vi "运维调试_采配水V4.vi"() -> ()   [LabVIEW 2016, in "PLC.lvlib"]
uses:
  PLC.lvlib
  control/switch.ctl
  <vilib>/Plasmionique/MB Master/MB_Master/MB_Master.lvclass
  <vilib>/Utility/miscctls.llb/LVPointTypeDef.ctl
  <vilib>/Plasmionique/MB Master/MB_Master_Serial/MB_Master_Serial.lvclass
  C:/Program Files (x86)/National Instruments/LabVIEW 2016/vi.lib/Plasmionique/MB Master/MB_Master/MB_Master.lvclass
  <vilib>/Instr/_visa.llb/VISA Configure Serial Port (Instr).vi
  <vilib>/Plasmionique/MB Master/MB Master.lvlib
panel:
  out "R135":i16 caption="除藻时间"
  in  "R134":u16(ring) caption="除藻工作模式" items=["手动", "自动"]
  in  "R110":u16(ring) caption="反冲洗水体" items=["自来水", "河水"]
  in  "63μm反冲洗阀":bool
  out "R34":u16
  in  "Y21":T1
  out "供水压力":dbl format="%.4f"
  out "R44":u16
  in  "Y31":T1
  out "R111":i16 caption="三级水样池润洗时间"
  in  "三级过滤系统":bool
  out "R104":i16 caption="三级润洗时间"
  out "R103":i16 caption="二级润洗时间"
  out "R107":i16 caption="进气时间"
  out "R43":u16
  in  "Y30":T1
  out "Registers":u16[](array[numeric])
  out "R124":i16 caption="加标回收配水时间"
  out "R42":i16
  in  "Y29":T1
  in  "更新程序":T1
  out "R122":i16 caption="二级自来水清洗时间"
  out "R121":i16 caption="一级自来水清洗时间"
  out "R120":i16 caption="过滤自来水清洗时间"
  out "清洗次数":u16
  out "当前启动泵号":u16(ring) items=["1号泵", "2号泵"]
  out "R116":i16 caption="储水时间"
  in  "R113":u16(ring) caption="水箱储水水体" items=["自来水", "河水"]
  out "R112":i16 caption="二级水样池进样超时"
  out "R31":u16
  out "R30":u16
  out "R29":u16
  out "R28":u16
  out "R27":u16
  out "R26":u16
  out "R25":u16
  out "R24":u16
  out "R23":u16
  out "R22":u16
  out "R21":u16
  out "R20":u16
  out "R19":u16
  out "R18":u16
  out "R17":u16
  out "R16":u16
  out "R15":u16
  out "R14":u16
  out "R13":u16
  out "配水压力":dbl format="%.4f"
  in  "Y18":T1
  in  "Y17":T1
  in  "Y14":T1
  in  "Y13":T1
  in  "Y1":T1
  in  "Y0":T1
  in  "Y12":T1
  in  "Y11":T1
  in  "Y10":T1
  in  "Y9":T1
  in  "Y8":T1
  in  "Y7":T1
  out "X2":bool caption="X1"
  out "采配水版本号":string
  out "R117":i16 caption="清洗频次设定"
  out "通讯故障":bool
  in  "R100":u16(ring) caption="采水泵工作模式" items=["泵1单泵单管路", "泵2单泵单管路", "潜水泵双泵双管路", "自吸泵双泵双管路"]
  out "X10":bool caption="氨氮水样池液位开关SL3"
  out "X9":bool caption="泵2过载报警_KM2"
  out "X8":bool caption="泵1过载报警_KM1"
  out "X7":bool caption="断电检测_PA"
  out "X6":bool caption="门禁开关_AS"
  out "X5":bool caption="烟雾检测_SA"
  out "X4":bool caption="浸水检测_WIA"
  out "X3":bool caption="水流开关_FS"
  out "X1":bool
  out "X0":bool caption="采样池液位开关_SL1"
  out "R109":i16 caption="外部反冲洗时间"
  out "集成报警信息":string
  out "R108":i16 caption="进样超时时间"
  out "R106":i16 caption="排液时间"
  out "R105":i16 caption="常规模式配水时间"
  out "R102":i16 caption="沉淀时间"
  out "R101":i16 caption="一级润洗时间"
  out "R2":i16
  out "R1":i16
  out "多列列表框":i32(listbox)
  in  "Y6":T1
  in  "Y5":T1
  in  "Y4":T1
  in  "Y3":T1
  in  "Y2":T1
  in  "Y16":T1
  in  "Y15":T1
  in  "返回":T1
  in  "参数设置":T1
  in  "单步启动":T1
  in  "启动":T1
  in  "停止":T1
  # "s"
  # "流程计时："
  # "s"
  # "单步计时："
  # "MPa"
  # "配水压力："
  # "MPa"
  # "供水压力："
  # "S"
  # "S"
  # "S"
  # "S"
  # "S"
  # "S"
  # "S"
  # "S"
  # "S"
  # "S"
  # "S"
  # "次"
  # "S"
  # "S"
  # "S"
  # "S"
  # "S"
  # "S"
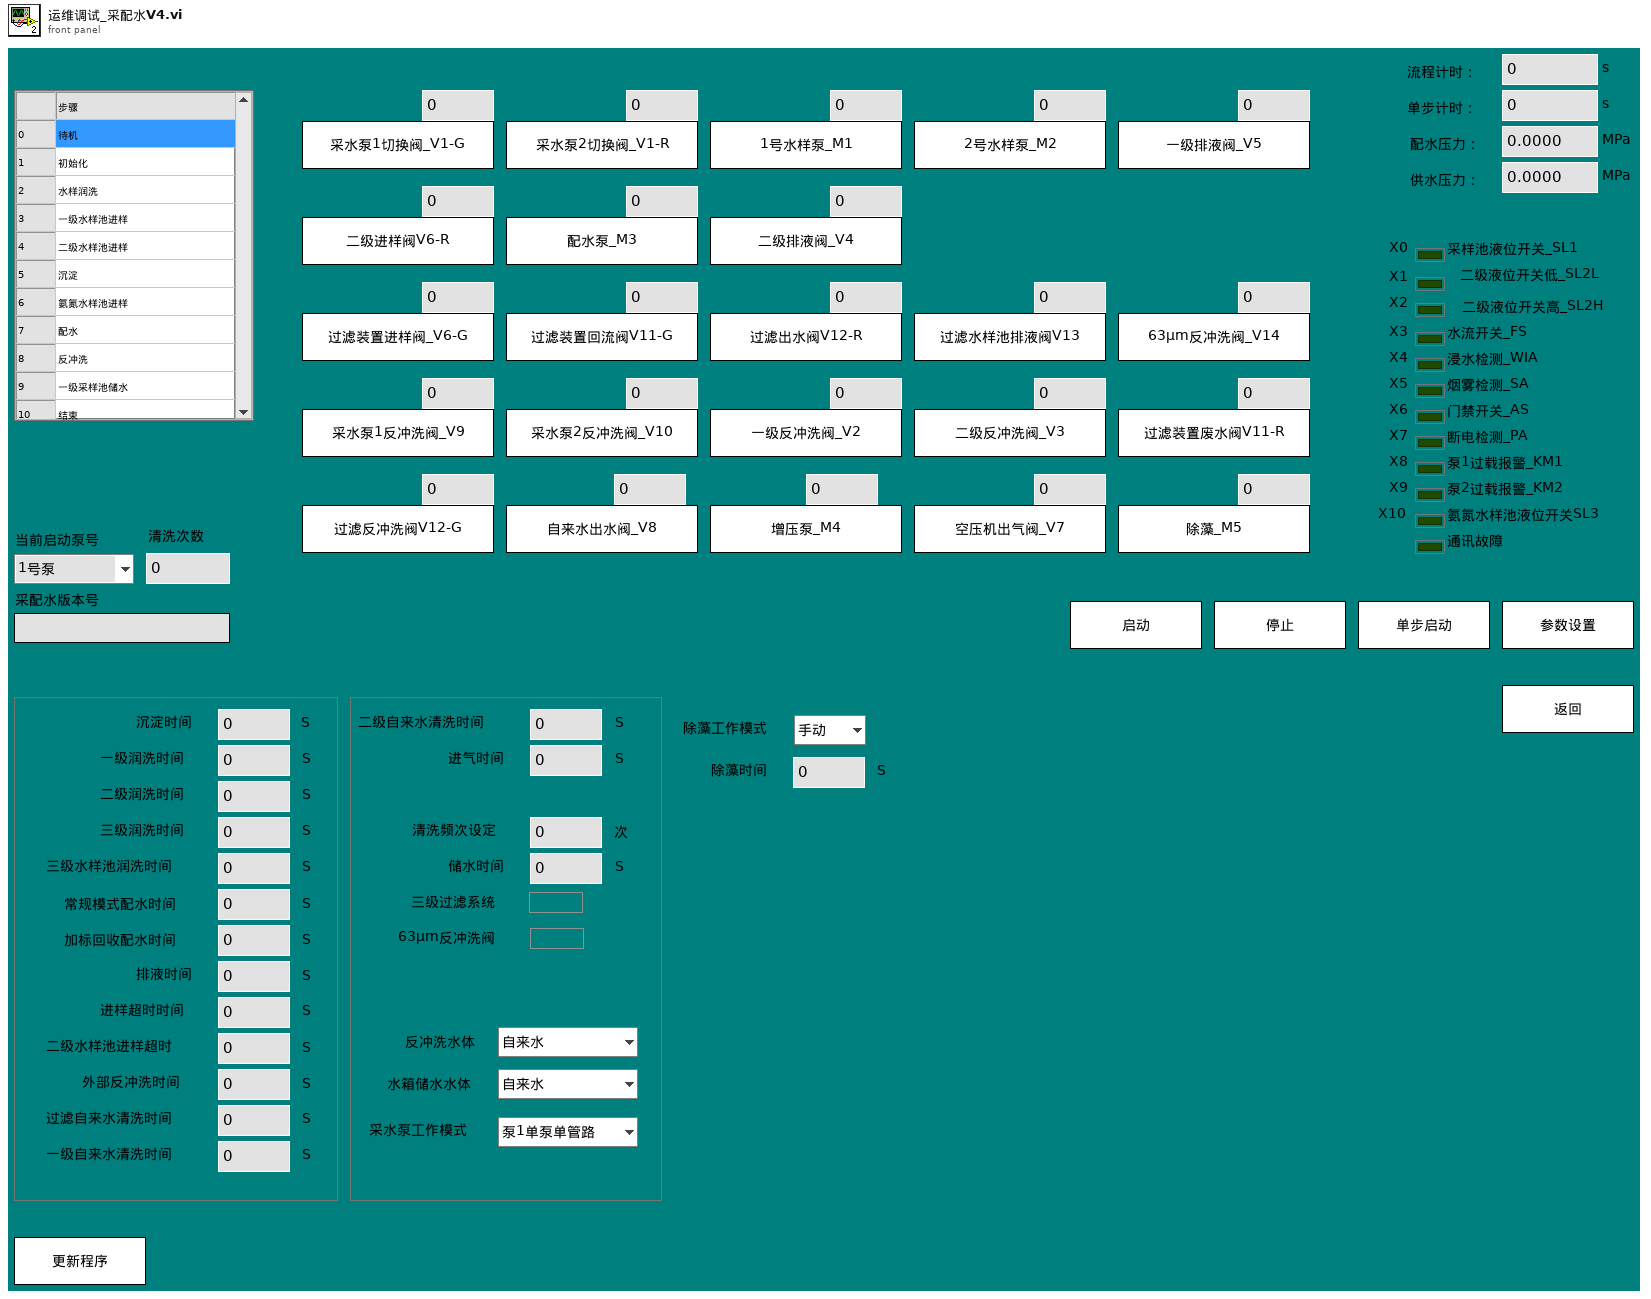
[diagram p1: front panel]
types:
  T1 = typedef "PLC.lvlib/switch.ctl" = bool
  T2 = typedef "参数.ctl" = cluster{"测试模式":enum16{"水样测试", "平行样测试", "集成干预测试", "加标回收"}, "参数启用":T3}
  T3 = typedef "启动参数.ctl" = cluster{"氨氮":bool, "总磷":bool, "总氮":bool, "多参数":bool, "CODmn":bool, "CODCr":bool, "氟化物":bool, "超标留样":bool, "重金属":bool, "挥发酚":bool}
  T4 = typedef "LVPointTypeDef.ctl" = cluster{"Horizontal":i16, "Vertical":i16}
  T5 = cluster{"命令":string, "数据":cluster{"starting address":u16, "holding register value":u16}}
  T6 = cluster{"R0":i16, "R1":i16, "R2":i16, "R3":i16, "R4":i16, "R5":i16, "R6":i16, "R7":i16, "R8":i16, "R9":i16, "R10":i16, "R11":i16, "R12":i16, "R13":i16, "R14":i16, "R15":i16, "R16":i16, "R17":i16, "R18":i16, "R19":i16, "R20":i16, "R21":i16, "R22":i16, "R23":i16, "R24":i16, "R25":i16, "R26":i16, "R27":i16, "R28":i16, "R29":i16, "R30":i16, "R31":i16, "R32":i16, "R33":i16, "R34":i16, "R35":i16, "R36":i16, "R37":i16, "R38":i16, "R39":i16, "R40":i16, "R41":i16, "R42":i16, "R43":i16, "R44":i16, "R45":i16, "R46":i16, "R47":i16, "R48":i16, "R49":i16, "R50":i16, "R51":i16, "R52":i16, "R53":i16, "R54":i16, "R55":i16, "R56":i16, "R57":i16, "R58":i16, "R59":i16, "R60":i16, "R61":i16, "R62":i16, "R63":i16, "R64":i16, "R65":i16, "R66":i16, "R67":i16, "R68":i16, "R69":i16, "R70":i16, "R71":i16, "R72":i16, "R73":i16, "R74":i16, "R75":i16, "R76":i16, "R77":i16, "R78":i16, "R79":i16}
  T7 = cluster{"seconds since 1Jan1904":timestamp, "table输入":string, string, "table输入":string}
  T8 = cluster{"命令":string, cluster{"starting address":u16, "holding register value":u16}}
  T9 = cluster{"命令":string, "数据":cluster{"starting address":u16, "holding register values":u16[]}}
  T10 = cluster{"命令":string, "data":cluster{"starting address":u16, "coil values":bool[]}}
  T11 = cluster{"测试模式":enum16{"水样测试", "平行样测试", "集成干预测试", "加标回收"}, "参数启用":T3}
  T12 = cluster{"baud rate (bps)":u32, "stop bits":u16, "parity":u16, "flow control":u16, "timeout":u32, "retries":i32}
  T13 = cluster{"starting address":u16, "holding register values":u16[]}
  T14 = cluster{"starting address":u16, "holding register value":u16}
  T15 = cluster{"starting address":u16, "coil values":bool[]}
  T16 = cluster{"Registers[0]":u16, "Registers[1]":u16, "Registers[2]":u16, "Registers[3]":u16, "Registers[4]":u16, "Registers[5]":u16, "Registers[6]":u16, "Registers[7]":u16, "Registers[8]":u16, "Registers[9]":u16, "Registers[10]":u16, "Registers[11]":u16, "Registers[12]":u16, "Registers[13]":u16, "Registers[14]":u16, "Registers[15]":u16, "Registers[16]":u16, "Registers[17]":u16, "Registers[18]":u16, "Registers[19]":u16, "Registers[20]":u16, "Registers[21]":u16, "Registers[22]":u16, "Registers[23]":u16, "Registers[24]":u16, "Registers[25]":u16, "Registers[26]":u16, "Registers[27]":u16, "Registers[28]":u16, "Registers[29]":u16, "Registers[30]":u16, "Registers[31]":u16, "Registers[32]":u16, "Registers[33]":u16, "Registers[34]":u16, "Registers[35]":u16, "Registers[36]":u16, "Registers[37]":u16, "Registers[38]":u16, "Registers[39]":u16, "Registers[40]":u16, "Registers[41]":u16, "Registers[42]":u16, "Registers[43]":u16, "Registers[44]":u16, "Registers[45]":u16, "Registers[46]":u16, "Registers[47]":u16, "Registers[48]":u16, "Registers[49]":u16, "Registers[50]":u16, "Registers[51]":u16, "Registers[52]":u16, "Registers[53]":u16, "Registers[54]":u16, "Registers[55]":u16, "Registers[56]":u16, "Registers[57]":u16, "Registers[58]":u16, "Registers[59]":u16, "Registers[60]":u16, "Registers[61]":u16, "Registers[62]":u16, "Registers[63]":u16, "Registers[64]":u16, "Registers[65]":u16, "Registers[66]":u16, "Registers[67]":u16, "Registers[68]":u16, "Registers[69]":u16, "Registers[70]":u16, "Registers[71]":u16, "Registers[72]":u16, "Registers[73]":u16, "Registers[74]":u16, "Registers[75]":u16, "Registers[76]":u16, "Registers[77]":u16, "Registers[78]":u16, "Registers[79]":u16}
  T17 = cluster{"Registers[0]":u16, "Registers[1]":u16, "Registers[2]":u16, "Registers[3]":u16, "Registers[4]":u16, "Registers[5]":u16}
  T18 = cluster{"Registers[0]":u16, "Registers[1]":u16, "Registers[2]":u16, "Registers[3]":u16, "Registers[4]":u16, "Registers[5]":u16, "Registers[6]":u16, "Registers[7]":u16, "Registers[8]":u16, "Registers[9]":u16, "Registers[10]":u16, "Registers[11]":u16, "Registers[12]":u16, "Registers[13]":u16, "Registers[14]":u16, "Registers[15]":u16, "Registers[16]":u16, "Registers[17]":u16, "Registers[18]":u16, "Registers[19]":u16, "Registers[20]":u16, "Registers[21]":u16, "Registers[22]":u16, "Registers[23]":u16, "Registers[24]":u16, "Registers[25]":u16, "Registers[26]":u16, "Registers[27]":u16, "Registers[28]":u16, "Registers[29]":u16, "Registers[30]":u16, "Registers[31]":u16, "Registers[32]":u16, "Registers[33]":u16, "Registers[34]":u16, "Registers[35]":u16}
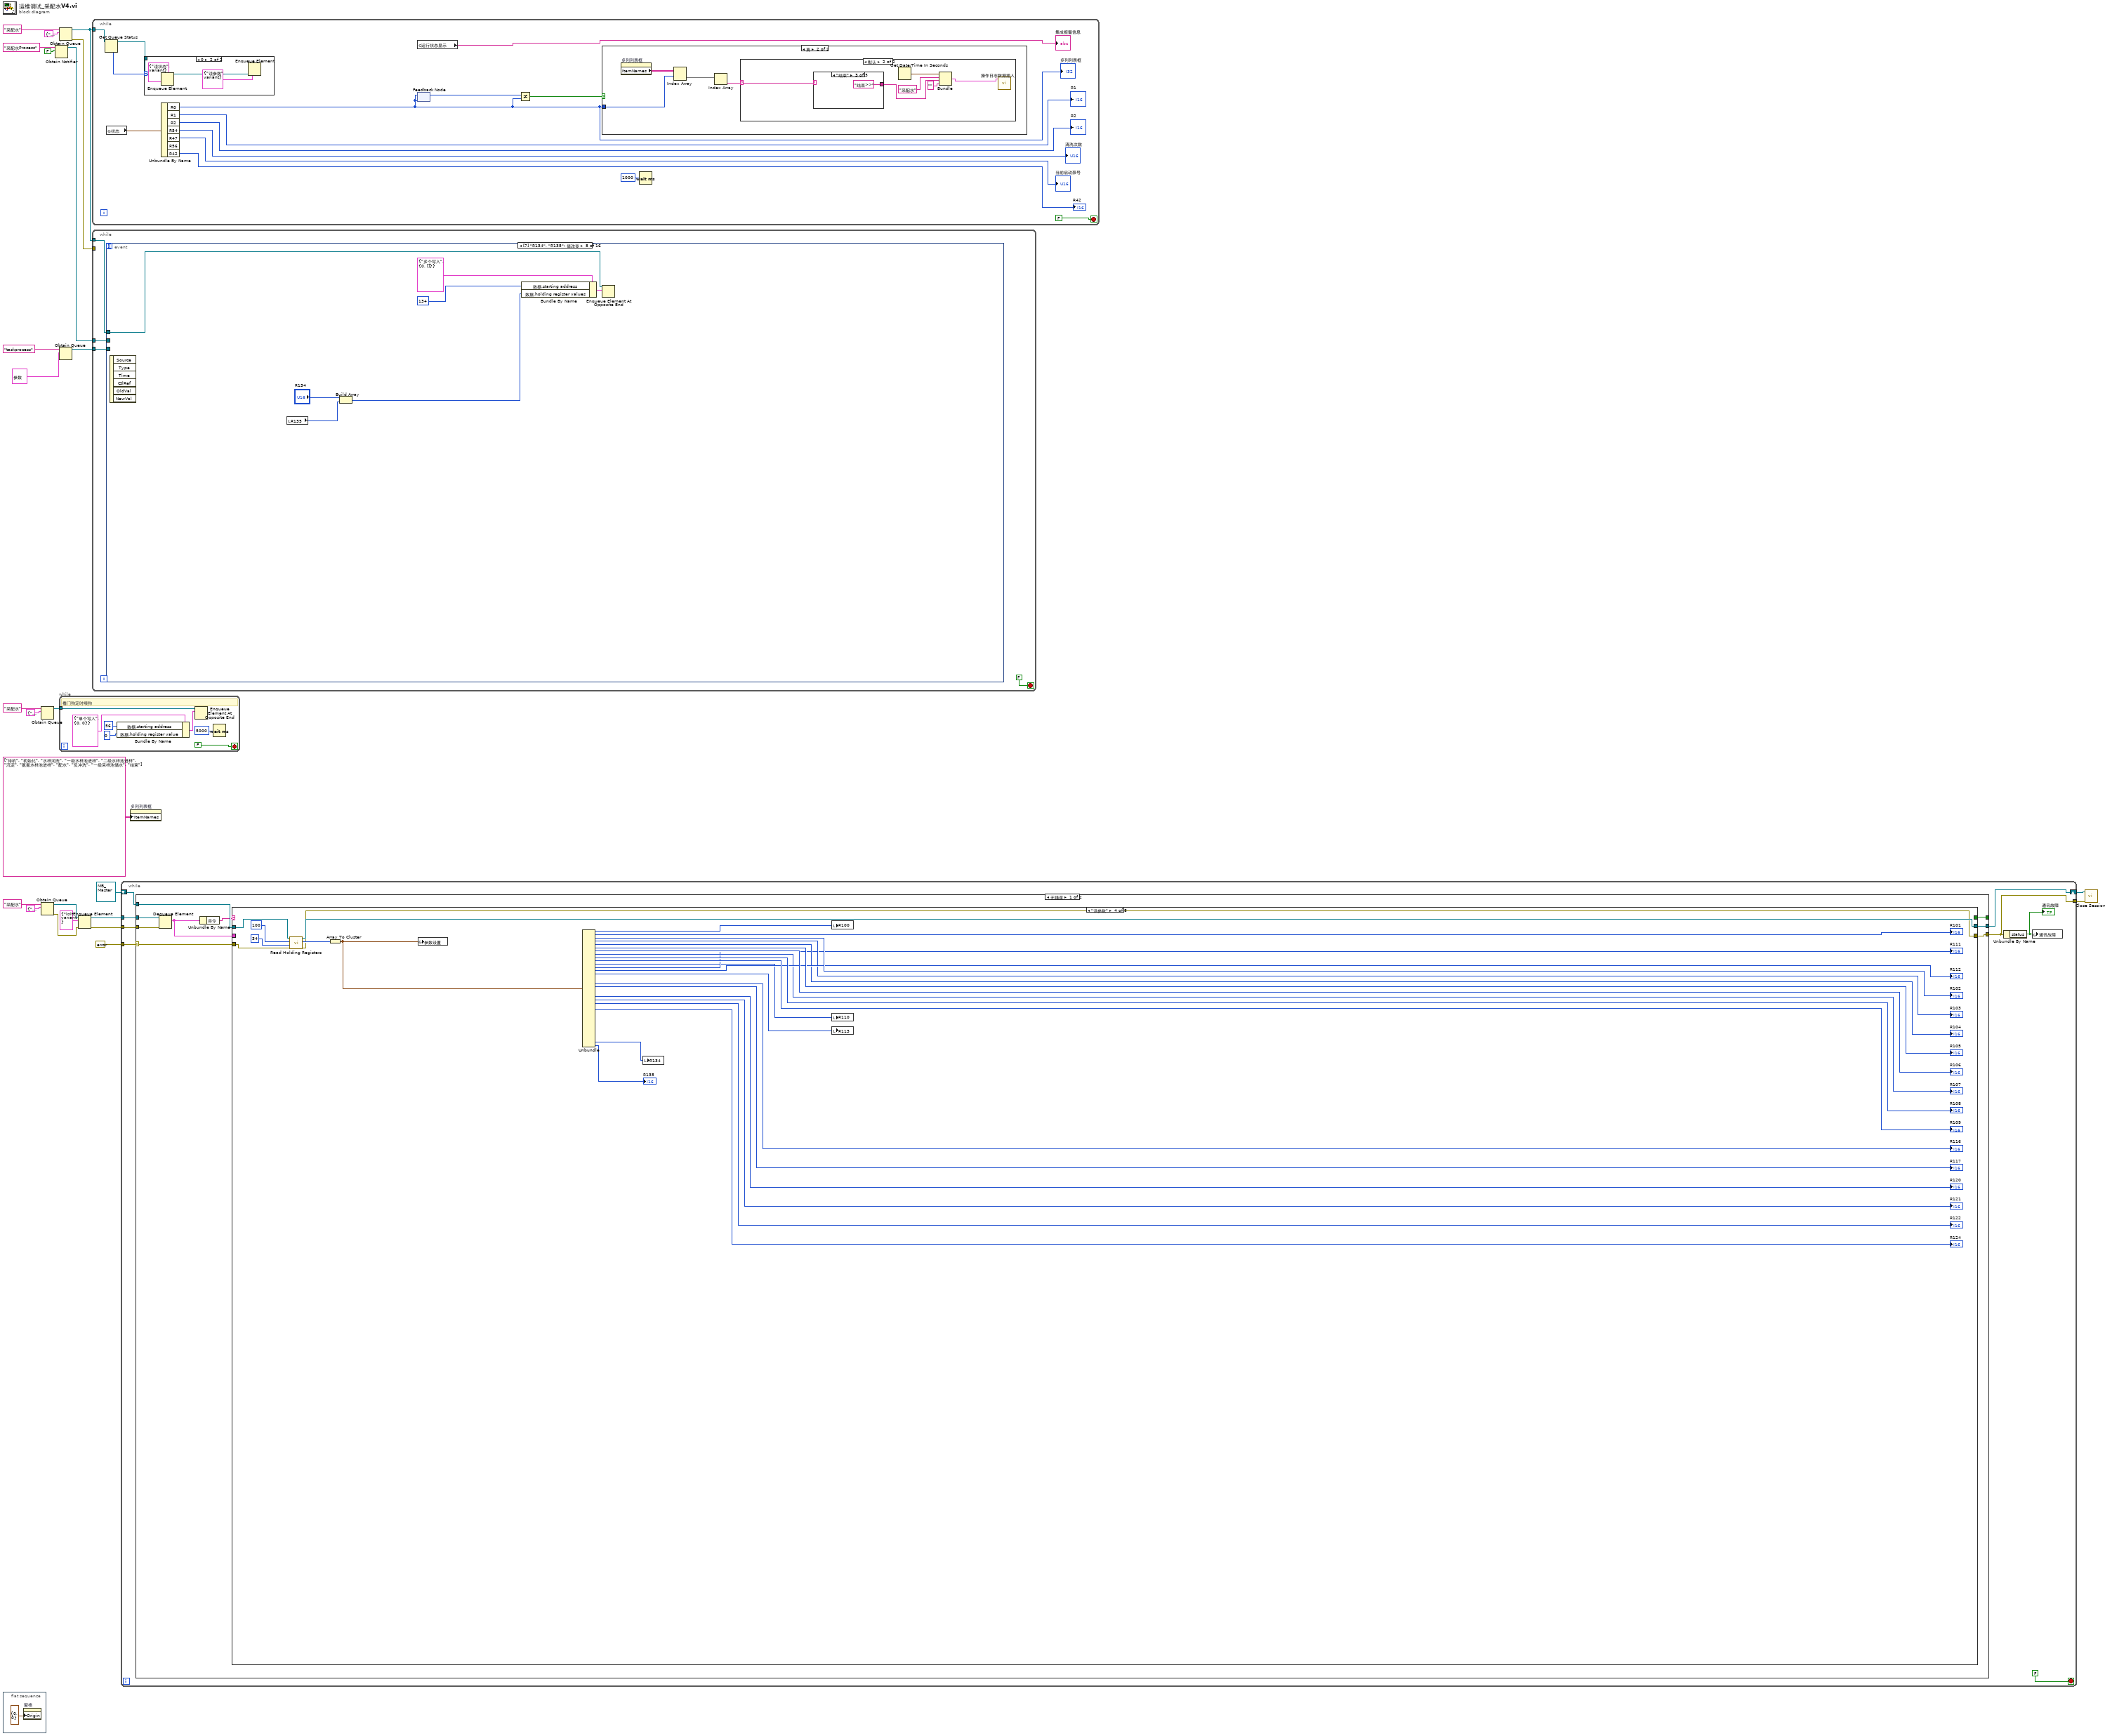
[diagram p0: block diagram]
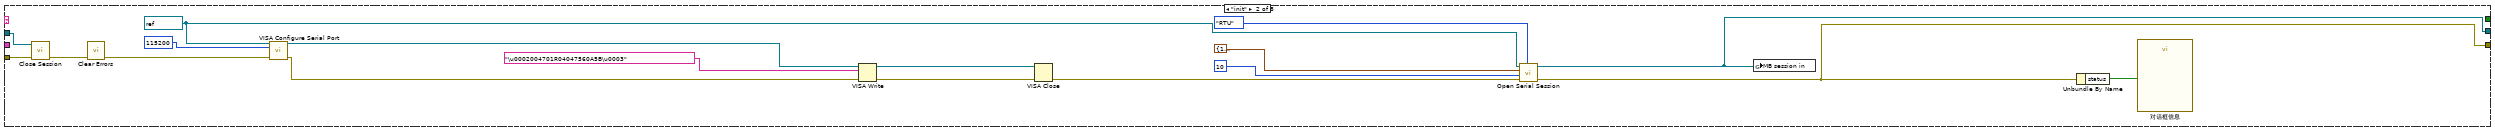
[diagram p3: hidden frame]
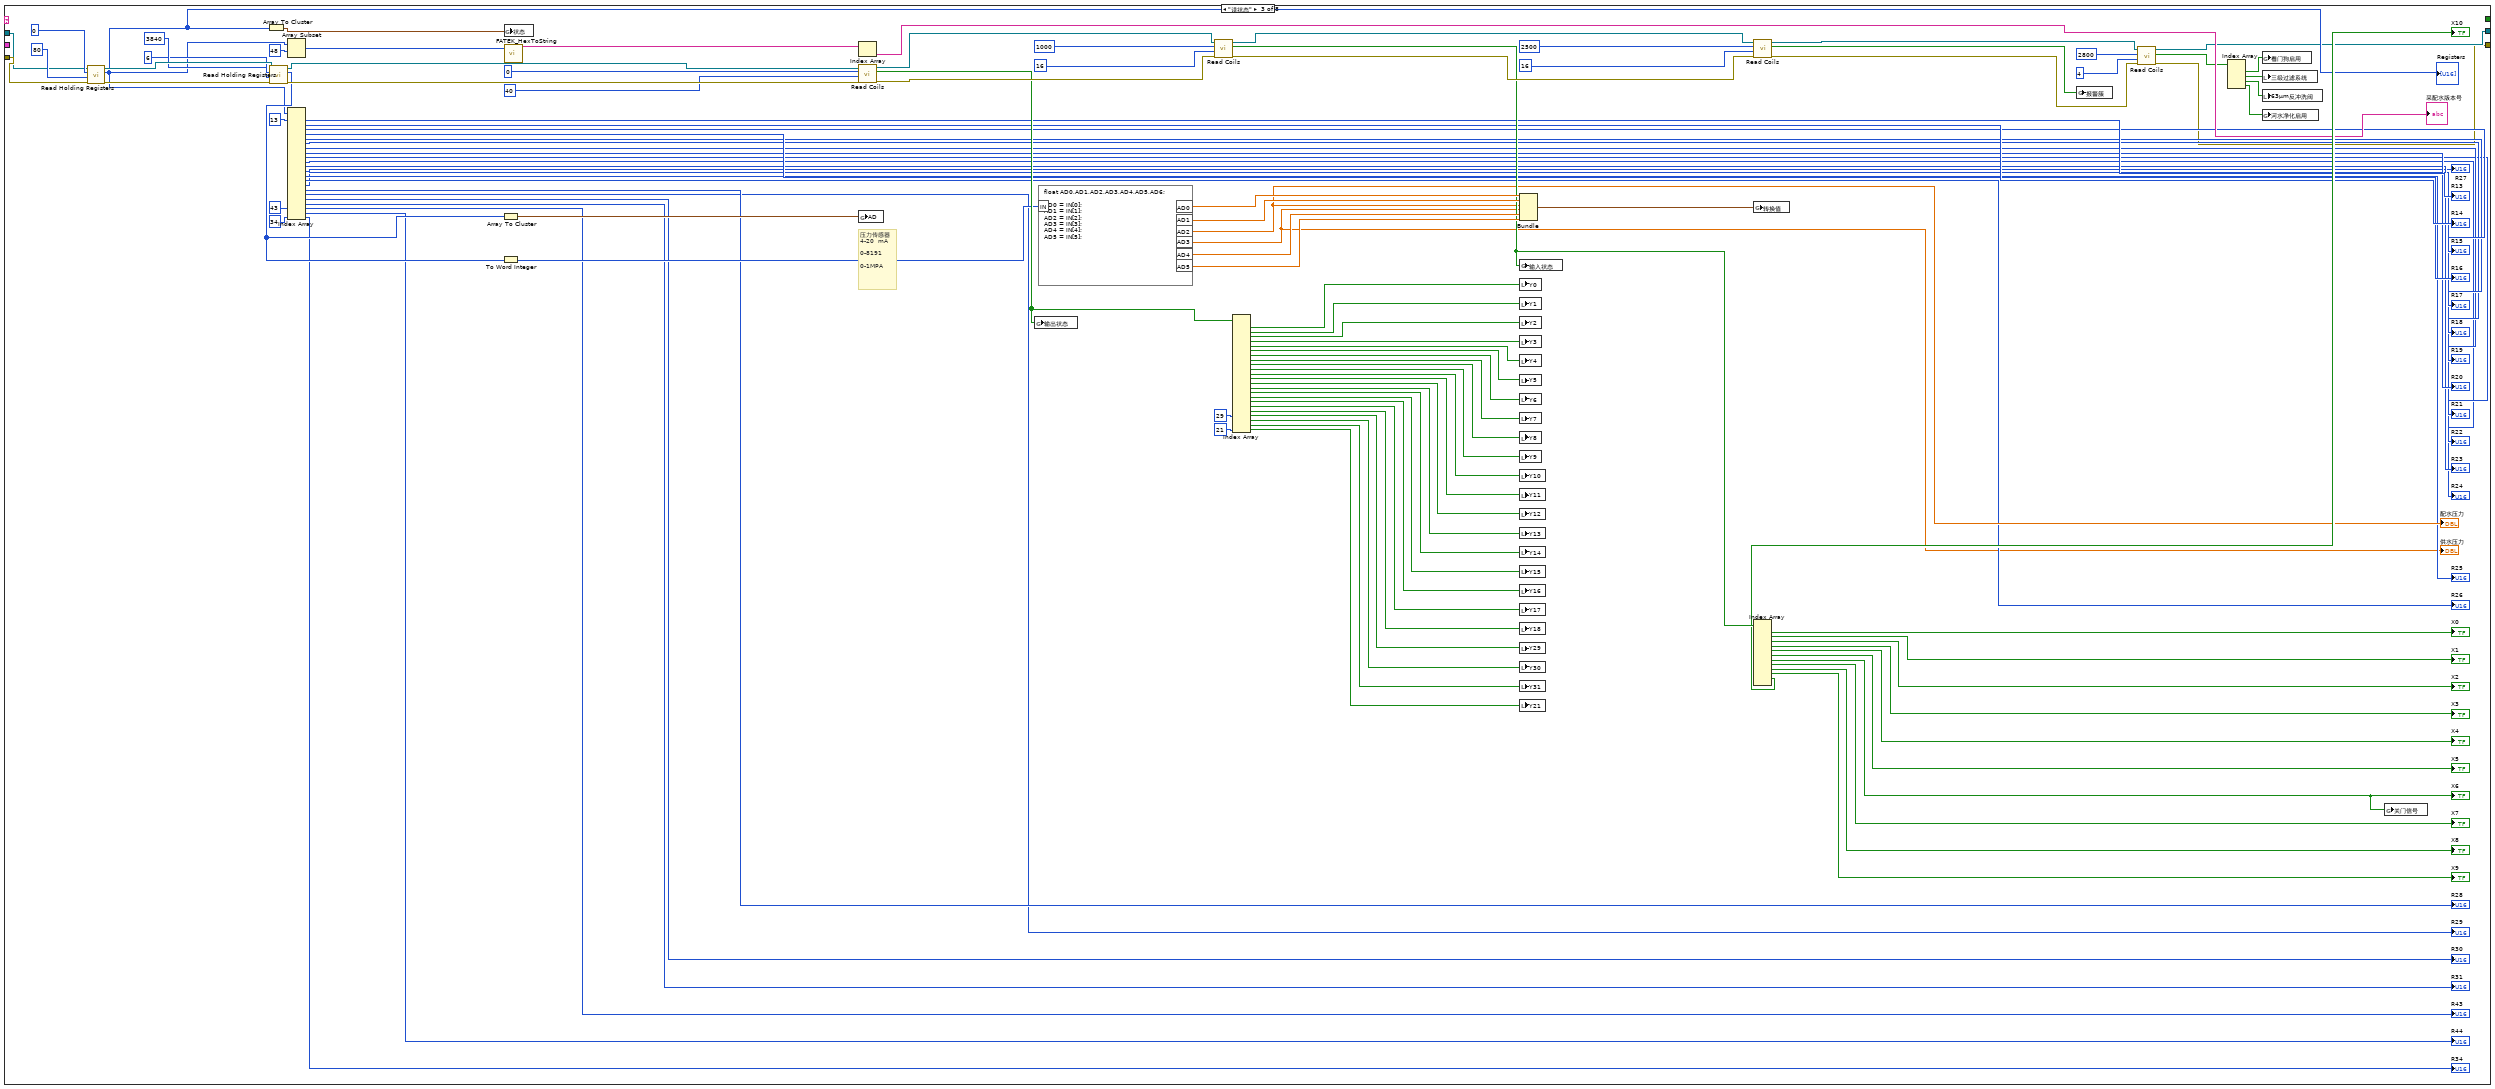
[diagram p4: hidden frame]
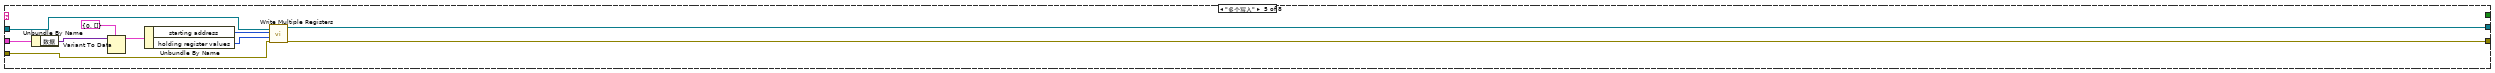
[diagram p5: hidden frame]
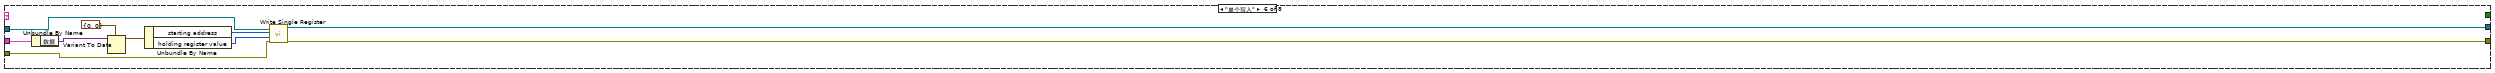
[diagram p6: hidden frame]
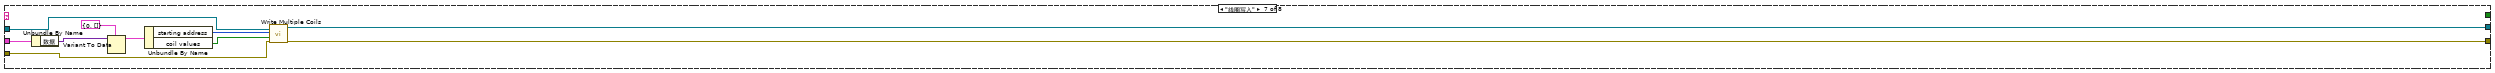
[diagram p7: hidden frame]
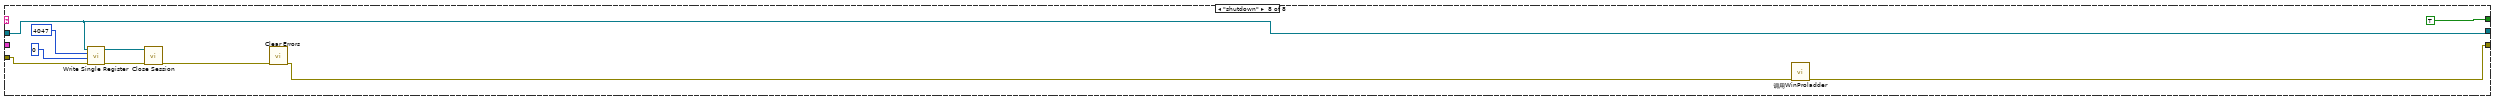
[diagram p8: hidden frame]
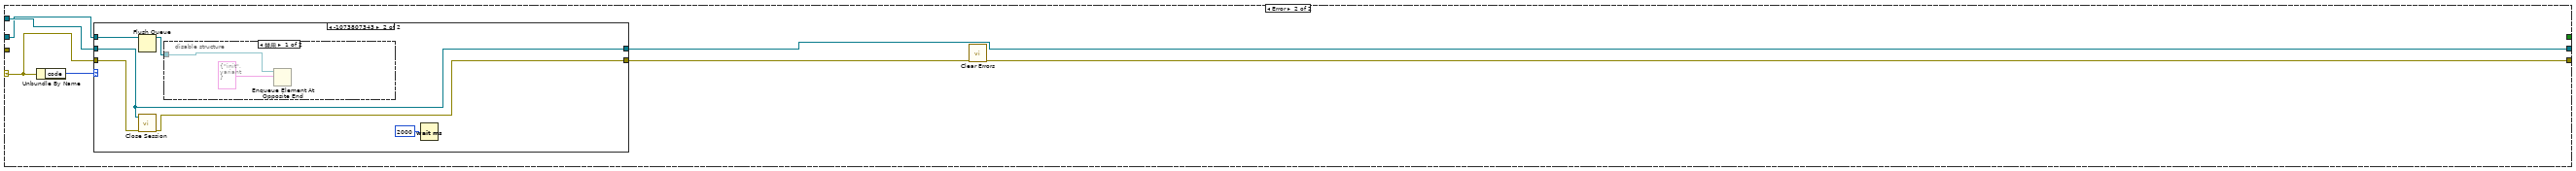
[diagram p9: hidden frame]
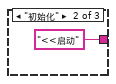
[diagram p16: hidden frame]
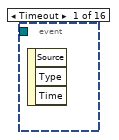
[diagram p17: hidden frame]
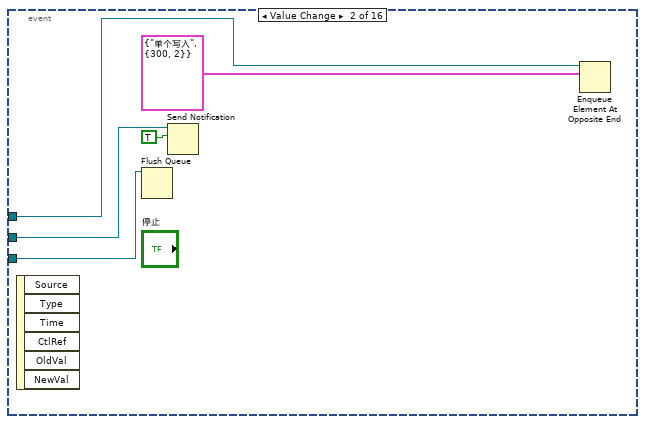
[diagram p18: hidden frame]
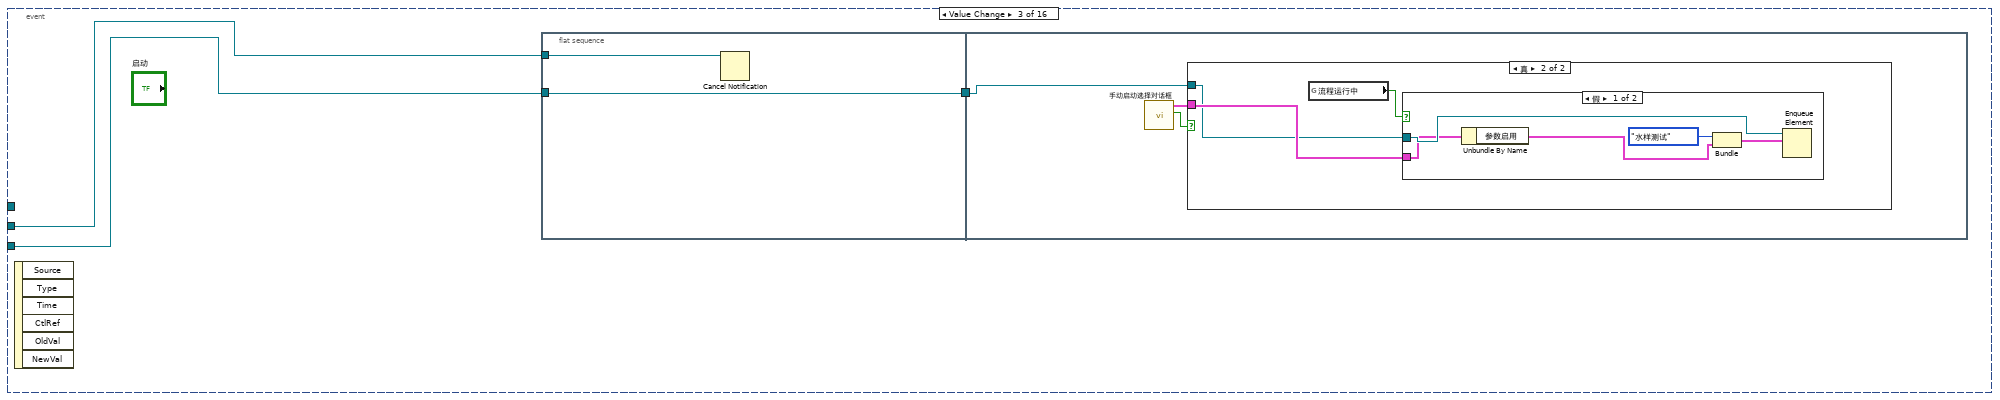
[diagram p19: hidden frame]
diagram:
  n1 = flat-sequence {
    frame #0 {
      n2 = property on="窗格" class="Pane"("Origin"=T4 {"Horizontal"=0, "Vertical"=0} ("原点")) -> ()  [unwired: 2 in, 2 out]
    }
  }
  n3 = Obtain Queue(name (unnamed)="采配水" ("名称（未命名）"), element data type=cluster{"命令":string, "数据":variant} {"命令"="", "数据"=variant}) -> (queue out=w4:refnum<queue>)  [unwired: 3 in, 2 out]
  n4 = Obtain Queue(name (unnamed)="采配水" ("名称（未命名）"), element data type=cluster{"命令":string, "数据":variant} {"命令"="", "数据"=variant}) -> (queue out=w15:refnum<queue>, error out=w14:errorcluster)  [unwired: 3 in, 1 out]
  n5 = Obtain Notifier(name (unnamed)="采配水Process" ("名称（未命名）"), notification data type=FALSE) -> (notifier out=w18:refnum<notifier>)  [unwired: 2 in, 2 out]
  n6 = while {
    tunnel: w4 -> [w31]
    stop <- FALSE stop-if-true
    # "看门狗定时喂狗"
    n7 = Bundle By Name(cluster=T5 {"命令"="单个写入", "数据"={"starting address"=0, "holding register value"=0}} ("元素"), "数据.starting address"=u16 56, "数据.holding register value"=u16 0) -> (w32:T5)
    n8 = Enqueue Element At Opposite End(queue=w31, element=w32) -> ()  [unwired: 2 in, 3 out]
    n9 = Wait (ms)(milliseconds to wait=u32 5000 ("等待时间（毫秒）")) -> ()  [unwired: 1 out]
  }
  n10 = Obtain Queue(name (unnamed)="采配水" ("名称（未命名）"), element data type=cluster{"命令":string, "数据":variant} {"命令"="", "数据"=variant}) -> (queue out=w22:refnum<queue>, error out=w23:errorcluster)  [unwired: 3 in, 1 out]
  n11 = Obtain Queue(name (unnamed)="taskprocess" ("名称（未命名）"), element data type=T2 {"测试模式"=enum."水样测试", "参数启用"={"氨氮"=FALSE, "总磷"=FALSE, "总氮"=FALSE, "多参数"=FALSE, "CODmn"=FALSE, "CODCr"=FALSE, "氟化物"=FALSE, "超标留样"=FALSE, "重金属"=FALSE, "挥发酚"=FALSE}} ("参数")) -> (queue out=w2:refnum<queue>)  [unwired: 3 in, 2 out]
  n12 = Enqueue Element(queue=w15, element=cluster{"命令":string, "数据":variant} {"命令"="init", "数据"=variant} ("元素"), error in (no error)=w14) -> (queue out=w10:refnum<queue>, error out=w12:errorcluster)  [unwired: 1 in, 1 out]
  n13 = while {
    tunnel: w22 -> [w47]
    stop <- FALSE stop-if-true
    n14 = Get Queue Status(queue=w47) -> (queue out=w35:refnum<queue>, # elements in queue=w34:i32)  [unwired: 2 in, 6 out]
    n15 = global read "采配水全局变量.vi" "状态"() -> (w46:T6)
    n16 = case shown="0" w34 {
      tunnel: w35 -> [_ w52]
      frame Default {
      }
      frame 0 {
        n17 = Enqueue Element(queue=w52, element=cluster{"命令":string, "数据":variant} {"命令"="读状态", "数据"=variant} ("元素")) -> (queue out=w49:refnum<queue>)  [unwired: 2 in, 2 out]
        n18 = Enqueue Element(queue=w49, element=cluster{"命令":string, "数据":variant} {"命令"="读参数", "数据"=variant} ("元素")) -> ()  [unwired: 2 in, 3 out]
      }
    }
    n19 = Unbundle By Name(w46) -> ("R0"=w39:i16, "R1"=→"R1":i16, "R2"=→"R2":i16, "R54"=→"清洗次数":i16, "R47"=→"当前启动泵号":i16, "R42"=→"R42":i16)  [unwired: 1 out]
    "多列列表框" <- w39
    n20 = global read "采配水全局变量.vi" "运行状态显示"() -> (→"集成报警信息":string)
    n21 = feedback-in #1(w39) -> ()
    n22 = feedback #1(w39) -> (w40:i16)
    n23 = Not Equal?(x=w40, y=w39) -> (x != y?=w43:bool)
    n24 = case shown="真" w43 {
      tunnel: w39 -> [_ w55]
      frame False {
      }
      frame True {
        n25 = property on="多列列表框" class="MCListbox (严格)"() -> ("ItemNames"=w56:string[][])  [unwired: 2 in, 2 out]
        n26 = Index Array(array=w56, index (row)=w55) -> (element=w54:string[])  [unwired: 1 in]
        n27 = Index Array(array=w54) -> (element=w53:string)  [unwired: 1 in]
        n28 = case shown="默认" w53 {
          selector: w53 -> [_ w59]
          frame "待机" {
          }
          frame Default {
            n29 = case shown="\"结束\"" w59 {
              selector: w59 -> [w63 _ _]
              tunnel: [w63 "<<启动" "结束>>"] -> w58
              frame Default {
              }
              frame "初始化" {
              }
              frame "结束" {
              }
            }
            n30 = Get Date/Time In Seconds() -> (seconds since 1Jan1904=w62:timestamp)
            n31 = Bundle("seconds since 1Jan1904"=w62, "table输入"="采配水", w58, "table输入"="") -> (w57:T7)  [unwired: 1 in]
            n32 = call "操作日志数据插入.vi"("data"=w57) -> ()  [unwired: 9 in, 1 out]
          }
        }
      }
    }
    n33 = Wait (ms)(milliseconds to wait=u32 1000 ("等待时间（毫秒）")) -> ()  [unwired: 1 out]
  }
  n34 = while {
    tunnel: w22 -> [w68]
    tunnel: w23 -> [_]
    tunnel: w18 -> [w67]
    tunnel: w2 -> [w66]
    stop <- FALSE stop-if-true
    n35 = event shown="[7] \"R134\", \"R135\": 值改变" {
      selector: _ -> [_ _ _ _ _ _ _ _ _ _ _ _ _ _ _ _]
      dyn-events: _ -> [_ _ _ _ _ _ _ _ _ _ _ _ _ _ _ _]
      timeout: _ -> [_ _ _ _ _ _ _ _ _ _ _ _ _ _ _ _]
      tunnel: w68 -> [_ w73 _ w95 w114 w123 w128 w135 _ _ _ w171 w174 w179 w184 w190]
      tunnel: w67 -> [_ w72 w77 _ _ _ _ _ _ _ _ _ _ _ _ _]
      tunnel: w66 -> [_ w70 w75 _ _ _ _ _ _ _ _ _ _ _ _ _]
      event Timeout {
        n36 = event-data() -> ()  [unwired: 1 in, 3 out]
      }
      event Value Change {
        n37 = event-data() -> ()  [unwired: 1 in, 6 out]
        n38 = Flush Queue(queue=w70) -> ()  [unwired: 1 in, 3 out]
        n39 = Send Notification(notification=TRUE ("通知"), notifier=w72) -> ()  [unwired: 1 in, 2 out]
        n40 = Enqueue Element At Opposite End(queue=w73, element=T8 {"命令"="单个写入", {"starting address"=300, "holding register value"=2}} ("元素")) -> ()  [unwired: 2 in, 3 out]
      }
      event Value Change {
        n41 = event-data() -> ()  [unwired: 1 in, 6 out]
        n42 = flat-sequence {
          tunnel: w77 -> [w79]
          tunnel: [w78] -> w76
          tunnel: w75 -> [w78]
          tunnel: w76 -> [w80]
          frame #0 {
            n43 = Cancel Notification(0:w79) -> ()  [unwired: 1 in, 3 out]
          }
          frame #1 {
            n44 = call "手动启动选择对话框.vi"() -> ("确定"=w82:bool, "输出簇"=w81:cluster{"参数启用":T3})  [unwired: 10 in]
            n45 = case shown="真" w82 {
              tunnel: w81 -> [_ w85]
              tunnel: w80 -> [_ w84]
              frame False {
              }
              frame True {
                n46 = global read "采配水全局变量.vi" "流程运行中"() -> (w83:bool)
                n47 = case shown="假" w83 {
                  tunnel: w85 -> [w88 _]
                  tunnel: w84 -> [w90 _]
                  frame False {
                    n48 = Unbundle By Name(w88) -> ("参数启用"=w87:T3)
                    n49 = Bundle("测试模式"=enum16{"水样测试", "平行样测试", "集成干预测试", "加标回收"}."水样测试", "参数启用"=w87) -> (w86:T11)  [unwired: 1 in]
                    n50 = Enqueue Element(queue=w90, element=w86) -> ()  [unwired: 2 in, 3 out]
                  }
                  frame True {
                    n51 = One Button Dialog(message="流程已启动，无需重复启动！" ("消息")) -> ()  [unwired: 1 in, 1 out]
                  }
                }
              }
            }
          }
        }
      }
      event Value Change {
        n52 = event-data() -> ()  [unwired: 1 in, 6 out]
        n53 = call "单步启动对话框.vi"() -> ("单步启动步骤输出"=w92:u16)  [unwired: 11 in]
        n54 = Bundle By Name(cluster=T5 {"命令"="单个写入", "数据"={"starting address"=301, "holding register value"=0}} ("元素"), "数据.holding register value"=w92) -> (w93:T5)
        n55 = Enqueue Element At Opposite End(queue=w95, element=w93) -> ()  [unwired: 2 in, 3 out]
      }
      event "R101", "R102", "R105", "R106", "R108", "R109", "R100", "R112", "R113", "R103", "R104", "R107", "R111", "R110": Value Change {
        n56 = event-data() -> ()  [unwired: 1 in, 6 out]
        n57 = local read "R101"() -> (w110:i16)
        n58 = local read "R102"() -> (w109:i16)
        n59 = local read "R103"() -> (w99:i16)
        n60 = local read "R104"() -> (w98:i16)
        n61 = local read "R105"() -> (w108:i16)
        n62 = local read "R106"() -> (w107:i16)
        n63 = local read "R107"() -> (w106:i16)
        n64 = local read "R108"() -> (w105:i16)
        n65 = local read "R109"() -> (w103:i16)
        n66 = local read "R111"() -> (w97:i16)
        n67 = local read "R112"() -> (w101:i16)
        n68 = Build Array("R100", w110, w109, w99, w98, w108, w107, w106, w105, w103, "R110", w97, w101, "R113") -> (w102:u16[])
        n69 = Bundle By Name(cluster=T9 {"命令"="多个写入", "数据"={"starting address"=0, "holding register values"=[]}} ("元素"), "数据.starting address"=u16 100, "数据.holding register values"=w102) -> (w111:T9)
        n70 = Enqueue Element At Opposite End(queue=w114, element=w111) -> ()  [unwired: 2 in, 3 out]
      }
      event "R116", "R117", "R120", "R121", "R122": Value Change {
        n71 = event-data() -> ()  [unwired: 1 in, 6 out]
        n72 = local read "R116"() -> (w121:i16)
        n73 = local read "R117"() -> (w120:i16)
        n74 = local read "R120"() -> (w119:i16)
        n75 = local read "R121"() -> (w118:i16)
        n76 = local read "R122"() -> (w117:i16)
        n77 = Build Array(w121, w120, i16 0 ("元素"), i16 0 ("R116"), w119, w118, w117) -> (w122:i16[])
        n78 = Bundle By Name(cluster=T9 {"命令"="多个写入", "数据"={"starting address"=0, "holding register values"=[]}} ("元素"), "数据.starting address"=u16 116, "数据.holding register values"=w122) -> (w124:T9)
        n79 = Enqueue Element At Opposite End(queue=w123, element=w124) -> ()  [unwired: 2 in, 3 out]
      }
      event "R124": Value Change {
        n80 = event-data() -> ("NewVal"=w127:i16)  [unwired: 1 in, 5 out]
        n81 = Build Array(w127) -> (w129:i16[])
        n82 = Bundle By Name(cluster=T9 {"命令"="多个写入", "数据"={"starting address"=0, "holding register values"=[]}} ("元素"), "数据.starting address"=u16 124, "数据.holding register values"=w129) -> (w130:T9)
        n83 = Enqueue Element At Opposite End(queue=w128, element=w130) -> ()  [unwired: 2 in, 3 out]
      }
      event "R134", "R135": Value Change {
        n84 = event-data() -> ()  [unwired: 1 in, 6 out]
        n85 = local read "R135"() -> (w133:i16)
        n86 = Build Array("R134", w133) -> (w136:u16[])
        n87 = Bundle By Name(cluster=T9 {"命令"="多个写入", "数据"={"starting address"=0, "holding register values"=[]}} ("元素"), "数据.starting address"=u16 134, "数据.holding register values"=w136) -> (w137:T9)
        n88 = Enqueue Element At Opposite End(queue=w135, element=w137) -> ()  [unwired: 2 in, 3 out]
      }
      event "R101", "R102", "R105", "R106", "R108", "R109", "R117", "R116", "R112", "R120", "R121", "R122", "R124", "R107", "R103", "R104", "R111", "R135": Mouse Down {
        n89 = event-data() -> ("CtlRef"=w143:refnum<vi>)  [unwired: 1 in, 7 out]
        n90 = property class="DigNum (严格)"(reference=w143) -> (reference out=w141:refnum<vi>, "Value"=w142:i16)  [unwired: 1 in, 1 out]
        n91 = call "数字键盘.vi"("OldNumber"=w142) -> ("NewNumber"=w140:sgl)
        n92 = property class="DigNum (严格)"(reference=w141, "Val(Sgnl)"=w140) -> ()  [unwired: 1 in, 2 out]
      }
      event Value Change {
        n93 = event-data() -> ()  [unwired: 1 in, 6 out]
        n94 = property on="窗格" class="Pane"("Origin"=T4 {"Horizontal"=0, "Vertical"=628} ("原点")) -> ()  [unwired: 2 in, 2 out]
      }
      event Value Change {
        n95 = event-data() -> ()  [unwired: 1 in, 6 out]
        n96 = property on="窗格" class="Pane"("Origin"=T4 {"Horizontal"=0, "Vertical"=0} ("原点")) -> ()  [unwired: 2 in, 2 out]
      }
      event Value Change {
        n97 = event-data() -> ()  [unwired: 1 in, 6 out]
        n98 = Build Array("Y0", "Y1", "Y2", "Y3", "Y4", "Y5", "Y6", "Y7", "Y8", "Y9", "Y10", "Y11", "Y12", "Y13", "Y14", "Y15", "Y16", "Y17", "Y18", "Y29", "Y30", "Y31") -> (w164:T1[])
        n99 = Bundle By Name(cluster=T10 {"命令"="线圈写入", "data"={"starting address"=2400, "coil values"=[]}} ("元素"), "data.coil values"=w164) -> (w165:T10)
        n100 = Enqueue Element(queue=w171, element=w165) -> ()  [unwired: 2 in, 3 out]
      }
      event Value Change {
        n101 = event-data() -> ()  [unwired: 1 in, 6 out]
        n102 = Build Array("Y21") -> (w172:T1[])
        n103 = Bundle By Name(cluster=T10 {"命令"="线圈写入", "data"={"starting address"=2451, "coil values"=[]}} ("元素"), "data.coil values"=w172) -> (w175:T10)
        n104 = Enqueue Element(queue=w174, element=w175) -> ()  [unwired: 2 in, 3 out]
      }
      event "三级过滤系统": Value Change {
        n105 = event-data() -> ()  [unwired: 1 in, 6 out]
        n106 = Build Array("三级过滤系统") -> (w177:bool[])
        n107 = Bundle By Name(cluster=T10 {"命令"="线圈写入", "data"={"starting address"=2801, "coil values"=[]}} ("元素"), "data.coil values"=w177) -> (w180:T10)
        n108 = Enqueue Element(queue=w179, element=w180) -> ()  [unwired: 2 in, 3 out]
      }
      event "63μm反冲洗阀": Value Change {
        n109 = event-data() -> ()  [unwired: 1 in, 6 out]
        n110 = Build Array("63μm反冲洗阀") -> (w183:bool[])
        n111 = Bundle By Name(cluster=T10 {"命令"="线圈写入", "data"={"starting address"=2802, "coil values"=[]}} ("元素"), "data.coil values"=w183) -> (w185:T10)
        n112 = Enqueue Element(queue=w184, element=w185) -> ()  [unwired: 2 in, 3 out]
      }
      event Value Change {
        n113 = event-data() -> ("NewVal"=w187:T1)  [unwired: 1 in, 5 out]
        n114 = Flush Queue(queue=w190) -> (queue out=w188:refnum<queue>)  [unwired: 1 in, 2 out]
        n115 = case shown="真" w187 {
          tunnel: [cluster{"命令":string, "数据":variant} {"命令"="init", "数据"=variant} ("元素") w194] -> w189
          frame False {
          }
          frame True {
            n116 = Two Button Dialog(message="警告，非专业人士请勿进行此操作！！！\n请确认是否释放串口？" ("消息")) -> (T button?=w193:bool)  [unwired: 2 in]
            n117 = case shown="真" w193 {
              tunnel: [_ cluster{"命令":string, "数据":variant} {"命令"="shutdown", "数据"=variant} ("元素")] -> w194
              frame False {
                n118 = local write "更新程序"(FALSE ("释放串口")) -> ()
              }
              frame True {
              }
            }
          }
        }
        n119 = Enqueue Element(queue=w188, element=w189) -> ()  [unwired: 2 in, 3 out]
      }
    }
  }
  n120 = while {
    tunnel: w10 -> [w201]
    tunnel: w12 -> [w200]
    shift-right: [w204] -> w7
    shift-left: refnum<class "MB_Master.lvclass"> refnum ("MB session in") -> [w203]
    tunnel: errorcluster {"status"=FALSE, "code"=0, "source"=""} ("error out") -> [w202]
    tunnel: [w199] -> w8
    stop <- FALSE stop-if-true
    n121 = case shown="无错误" w202 {
      selector: w202 -> [w210 w419]
      tunnel: [w213 w418] -> w204
      tunnel: w203 -> [w212 w420]
      tunnel: [w211 w416] -> w199
      tunnel: w201 -> [w207 w415]
      tunnel: w200 -> [w206 _]
      tunnel: [w208 _] -> _
      frame No Error {
        n122 = Dequeue Element(queue=w207, error in (no error)=w206) -> (element=w205:cluster{"命令":string, "数据":variant})  [unwired: 1 in, 3 out]
        n123 = Unbundle By Name(w205) -> ("命令"=w209:string)
        n124 = case shown="\"读参数\"" w209 {
          tunnel: [w215 w216 w254 w369 w381 w391 w401 w412] -> w213
          tunnel: w212 -> [w215 w230 w335 w374 w384 w394 w404 w412]
          tunnel: [w214 w229 w244 w368 w382 w392 w402 w405] -> w211
          tunnel: w210 -> [w214 w232 w338 w373 w383 w393 w403 w408]
          tunnel: [_ _ _ _ _ _ _ TRUE] -> w208
          tunnel: w205 -> [_ _ _ _ w380 w390 w400 _]
          frame "idle", Default {
          }
          frame "init" {
            w220 = refnum<visa-resource-name> "COM3" ("VISA resource name")
            n125 = call-dynamic "Close Session.vi"("error in (no error)"=w232, "MB session in"=w230) -> ("error out"=w231:errorcluster)  [unwired: 9 in]
            n126 = call <vilib>:"Clear Errors.vi"("error in (no error)"=w231) -> ("error out"=w218:errorcluster)  [unwired: 5 in, 1 out]
            n127 = call-poly "VISA Configure Serial Port"("VISA resource name"=w220, "baud rate (9600)"=u32 115200, "error in (no error)"=w218) -> ("VISA resource name out"=w225:refnum<visa-resource-name>, "error out"=w224:errorcluster)  [unwired: 11 in]
            n128 = VISA Write(VISA resource name=w225, write buffer="\u0002004701R04047560A5B\u0003" ("写入缓冲区"), error in (no error)=w224) -> (VISA resource name out=w223:refnum<visa-resource-name>, error out=w222:errorcluster)  [unwired: 1 out]
            n129 = VISA Close(VISA resource name=w223, error in (no error)=w222) -> (error out=w217:errorcluster)
            n130 = call <vilib>:"Open Serial Session.vi"("Mode (RTU)"=enum16{"RTU", "ASCII"}."RTU", "Error in"=w217, "Slave ID"=u8 10, "Serial Config"=T12 {"baud rate (bps)"=115200, "stop bits"=10, "parity"=0, "flow control"=0, "timeout"=500, "retries"=1}, "VISA Resource"=w220) -> ("Error out"=w229:errorcluster, "MB_Serial session"=w216:refnum<class "MB_Master_Serial.lvclass">)  [unwired: 5 in]
            n131 = global write "采配水全局变量.vi" "MB session in"(w216) -> ()
            n132 = Unbundle By Name(w229) -> ("status"=w233:bool)
            n133 = call "对话框信息"("Enable"=w233) -> ()  [unwired: 9 in, 2 out]
          }
          frame "读状态" {
            # "压力传感器\n4-20  mA \n \n0-8191\n\n0-1MPA"
            n134 = call <vilib>:"Read Holding Registers.vi"("error in (no error)"=w338, "quantity"=u16 80 ("number of holding registers"), "starting address"=u16 0, "MB session in"=w335) -> ("error out"=w333:errorcluster, "Registers"=w279:u16[], "MB session out"=w334:refnum<class "MB_Master.lvclass">)  [unwired: 5 in]
            "Registers" <- w279
            n135 = Array To Cluster(array=w279) -> (cluster=w258:T16)
            n136 = call <vilib>:"Read Holding Registers.vi"("error in (no error)"=w333, "quantity"=u16 6 ("number of holding registers"), "starting address"=u16 3840, "MB session in"=w334) -> ("error out"=w329:errorcluster, "Registers"=w308:u16[], "MB session out"=w330:refnum<class "MB_Master.lvclass">)  [unwired: 5 in]
            n137 = Array Subset(array=w279, index=48 ("索引")) -> (w305:u16[])  [unwired: 1 in]
            n138 = Index Array(array=w279, index #1=13 ("索引"), index #20=43 ("索引"), index #22=34 ("索引")) -> (element #1=→"R13":u16, element #2=→"R14":u16, element #3=→"R15":u16, element #4=→"R16":u16, element #5=→"R17":u16, element #6=→"R18":u16, element #7=→"R19":u16, element #8=→"R20":u16, element #9=→"R21":u16, element #10=→"R22":u16, element #11=→"R23":u16, element #12=→"R24":u16, element #13=→"R25":u16, element #14=→"R26":u16, element #15=→"R27":u16, element #16=→"R28":u16, element #17=→"R29":u16, element #18=→"R30":u16, element #19=→"R31":u16, element #20=→"R43":u16, element #21=→"R44":u16, element #22=→"R34":u16)  [unwired: 19 in]
            n139 = Array To Cluster(array=w308) -> (cluster=w344:T17)
            n140 = To Word Integer(number=w308) -> (16bit integer=w307:i16[])
            n141 = global write "采配水全局变量.vi" "状态"(w258) -> ()
            n142 = call "FATEK_HexToString.vi"("数组"=w305) -> ("STRING"=w304:string[])  [unwired: 10 in]
            n143 = Index Array(array=w304) -> (element=→"采配水版本号":string)  [unwired: 1 in]
            n144 = call <vilib>:"Read Coils.vi"("error in (no error)"=w329, "quantity"=u16 40 ("number of coils"), "starting address"=u16 0, "MB session in"=w330) -> ("error out"=w325:errorcluster, "Coils"=w311:bool[], "MB session out"=w326:refnum<class "MB_Master.lvclass">)  [unwired: 5 in]
            n145 = global write "采配水全局变量.vi" "AD"(w344) -> ()
            n146 = global write "采配水全局变量.vi" "输出状态"(w311) -> ()
            n147 = formula code="float AD0,AD1,AD2,AD3,AD4,AD5,AD6;\n\nAD0 = IN[0];\nAD1 = IN[1];\nAD2 = IN[2];\nAD3 = IN[3];\nAD4 = IN[4];\nAD5 = IN[5];"("IN"=w307) -> ("AD0"=w342:dbl, "AD1"=w341:dbl, "AD2"=w287:dbl, "AD3"=w241:dbl, "AD4"=w340:dbl, "AD5"=w339:dbl)
            "配水压力" <- w287
            "供水压力" <- w241
            n148 = call <vilib>:"Read Coils.vi"("error in (no error)"=w325, "quantity"=u16 16 ("number of coils"), "starting address"=u16 1000, "MB session in"=w326) -> ("error out"=w321:errorcluster, "Coils"=w317:bool[], "MB session out"=w322:refnum<class "MB_Master.lvclass">)  [unwired: 5 in]
            n149 = Index Array(array=w311, index #20=29 ("索引"), index #23=21 ("索引")) -> (element #1=w286:bool, element #2=w302:bool, element #3=w301:bool, element #4=w300:bool, element #5=w299:bool, element #6=w298:bool, element #7=w297:bool, element #8=w293:bool, element #9=w292:bool, element #10=w291:bool, element #11=w290:bool, element #12=w289:bool, element #13=w288:bool, element #14=w285:bool, element #15=w284:bool, element #16=w283:bool, element #17=w282:bool, element #18=w281:bool, element #19=w280:bool, element #20=w256:bool, element #21=w249:bool, element #22=w243:bool, element #23=w237:bool)  [unwired: 21 in]
            n150 = Bundle(w342, w341, w287, w241, w340, w339) -> (w343:cluster{dbl, dbl, dbl, dbl, dbl, dbl})  [unwired: 1 in]
            n151 = global write "采配水全局变量.vi" "输入状态"(w317) -> ()
            n152 = local write "Y0"(w286) -> ()
            n153 = local write "Y1"(w302) -> ()
            n154 = local write "Y2"(w301) -> ()
            n155 = local write "Y3"(w300) -> ()
            n156 = local write "Y4"(w299) -> ()
            n157 = local write "Y5"(w298) -> ()
            n158 = local write "Y6"(w297) -> ()
            n159 = local write "Y7"(w293) -> ()
            n160 = local write "Y8"(w292) -> ()
            n161 = local write "Y9"(w291) -> ()
            n162 = local write "Y10"(w290) -> ()
            n163 = local write "Y11"(w289) -> ()
            n164 = local write "Y12"(w288) -> ()
            n165 = local write "Y13"(w285) -> ()
            n166 = local write "Y14"(w284) -> ()
            n167 = local write "Y15"(w283) -> ()
            n168 = local write "Y16"(w282) -> ()
            n169 = local write "Y17"(w281) -> ()
            n170 = local write "Y18"(w280) -> ()
            n171 = local write "Y29"(w256) -> ()
            n172 = local write "Y30"(w249) -> ()
            n173 = local write "Y31"(w243) -> ()
            n174 = local write "Y21"(w237) -> ()
            n175 = call <vilib>:"Read Coils.vi"("error in (no error)"=w321, "quantity"=u16 16 ("number of coils"), "starting address"=u16 2500, "MB session in"=w322) -> ("error out"=w245:errorcluster, "Coils"=w318:bool[], "MB session out"=w255:refnum<class "MB_Master.lvclass">)  [unwired: 5 in]
            n176 = global write "采配水全局变量.vi" "转换值"(w343) -> ()
            n177 = Index Array(array=w317) -> (element #1=→"X0":bool, element #2=→"X1":bool, element #3=→"X2":bool, element #4=→"X3":bool, element #5=→"X4":bool, element #6=→"X5":bool, element #7=w234:bool, element #8=→"X7":bool, element #9=→"X8":bool, element #10=→"X9":bool, element #11=→"X10":bool)  [unwired: 12 in, 1 out]
            "X6" <- w234
            n178 = global write "采配水全局变量.vi" "报警簇"(w318) -> ()
            n179 = call <vilib>:"Read Coils.vi"("error in (no error)"=w245, "quantity"=u16 4, "starting address"=u16 2800, "MB session in"=w255) -> ("error out"=w244:errorcluster, "Coils"=w251:bool[], "MB session out"=w254:refnum<class "MB_Master.lvclass">)  [unwired: 5 in]
            n180 = Index Array(array=w251) -> (element #1=w250:bool, element #2=w246:bool, element #3=w236:bool, element #4=w235:bool)  [unwired: 4 in]
            n181 = global write "采配水全局变量.vi" "看门狗启用"(w250) -> ()
            n182 = local write "三级过滤系统"(w246) -> ()
            n183 = local write "63μm反冲洗阀"(w236) -> ()
            n184 = global write "采配水全局变量.vi" "河水净化启用"(w235) -> ()
            n185 = global write "采配水全局变量.vi" "关门信号"(w234) -> ()
          }
          frame "读参数" {
            n186 = call <vilib>:"Read Holding Registers.vi"("error in (no error)"=w373, "quantity"=u16 34 ("number of holding registers"), "starting address"=u16 100, "MB session in"=w374) -> ("error out"=w368:errorcluster, "Registers"=w370:u16[], "MB session out"=w369:refnum<class "MB_Master.lvclass">)  [unwired: 5 in]
            n187 = Array To Cluster(array=w370) -> (cluster=w361:T18)
            n188 = global write "采配水全局变量.vi" "参数设置"(w361) -> ()
            n189 = Unbundle(w361) -> ("Registers[0]"=w360:u16, "Registers[1]"=→"R101":u16, "Registers[2]"=→"R102":u16, "Registers[3]"=→"R103":u16, "Registers[4]"=→"R104":u16, "Registers[5]"=→"R105":u16, "Registers[6]"=→"R106":u16, "Registers[7]"=→"R107":u16, "Registers[8]"=→"R108":u16, "Registers[9]"=→"R109":u16, "Registers[10]"=w347:u16, "Registers[11]"=→"R111":u16, "Registers[12]"=→"R112":u16, "Registers[13]"=w357:u16, "Registers[16]"=→"R116":u16, "Registers[17]"=→"R117":u16, "Registers[20]"=→"R120":u16, "Registers[21]"=→"R121":u16, "Registers[22]"=→"R122":u16, "Registers[24]"=→"R124":u16, "Registers[34]"=w345:u16, "Registers[35]"=→"R135":u16)  [unwired: 14 out]
            n190 = local write "R134"(w345) -> ()
            n191 = local write "R100"(w360) -> ()
            n192 = local write "R110"(w347) -> ()
            n193 = local write "R113"(w357) -> ()
          }
          frame "多个写入" {
            n194 = Unbundle By Name(w380) -> ("数据"=w379:variant)
            n195 = Variant To Data(type=T13 {"starting address"=0, "holding register values"=[]}, Variant=w379) -> (data=w377:T13)  [unwired: 1 in, 1 out]
            n196 = Unbundle By Name(w377) -> ("starting address"=w376:u16, "holding register values"=w375:u16[])
            n197 = call <vilib>:"Write Multiple Registers.vi"("error in (no error)"=w383, "values"=w375, "starting address"=w376, "MB session in"=w384) -> ("error out"=w382:errorcluster, "MB session out"=w381:refnum<class "MB_Master.lvclass">)  [unwired: 6 in]
          }
          frame "单个写入" {
            n198 = Unbundle By Name(w390) -> ("数据"=w389:variant)
            n199 = Variant To Data(type=T14 {"starting address"=0, "holding register value"=0}, Variant=w389) -> (data=w387:T14)  [unwired: 1 in, 1 out]
            n200 = Unbundle By Name(w387) -> ("starting address"=w386:u16, "holding register value"=w385:u16)
            n201 = call <vilib>:"Write Single Register.vi"("error in (no error)"=w393, "value"=w385, "address"=w386, "MB session in"=w394) -> ("error out"=w392:errorcluster, "MB session out"=w391:refnum<class "MB_Master.lvclass">)  [unwired: 6 in]
          }
          frame "线圈写入" {
            n202 = Unbundle By Name(w400) -> ("数据"=w399:variant)
            n203 = Variant To Data(type=T15 {"starting address"=0, "coil values"=[]}, Variant=w399) -> (data=w397:T15)  [unwired: 1 in, 1 out]
            n204 = Unbundle By Name(w397) -> ("starting address"=w396:u16, "coil values"=w395:bool[])
            n205 = call <vilib>:"Write Multiple Coils.vi"("error in (no error)"=w403, "values"=w395, "starting address"=w396, "MB session in"=w404) -> ("error out"=w402:errorcluster, "MB session out"=w401:refnum<class "MB_Master.lvclass">)  [unwired: 6 in]
          }
          frame "shutdown" {
            n206 = call <vilib>:"Write Single Register.vi"("error in (no error)"=w408, "value"=u16 0, "address"=u16 4047, "MB session in"=w412) -> ("error out"=w407:errorcluster, "MB session out"=w411:refnum<class "MB_Master.lvclass">)  [unwired: 6 in]
            n207 = call-dynamic "Close Session.vi"("error in (no error)"=w407, "MB session in"=w411) -> ("error out"=w413:errorcluster)  [unwired: 9 in]
            n208 = call <vilib>:"Clear Errors.vi"("error in (no error)"=w413) -> ("error out"=w406:errorcluster)  [unwired: 5 in, 1 out]
            n209 = call "调用WinProladder.vi"("错误输入（无错误）"=w406) -> ("错误输出"=w405:errorcluster)  [unwired: 10 in]
          }
        }
      }
      frame Error {
        n210 = Unbundle By Name(w419) -> ("code"=w421:i32)
        n211 = case shown="-1073807343" w421 {
          tunnel: w420 -> [w423 w427]
          tunnel: w419 -> [w422 w429]
          tunnel: [w422 w428] -> w417
          tunnel: [w423 w427] -> w418
          tunnel: w415 -> [_ w426]
          frame Default {
          }
          frame -1073807343 {
            n212 = Flush Queue(queue=w426) -> (queue out=w425:refnum<queue>)  [unwired: 1 in, 2 out]
            n213 = call-dynamic "Close Session.vi"("error in (no error)"=w429, "MB session in"=w427) -> ("error out"=w428:errorcluster)  [unwired: 9 in]
            n214 = disable-structure shown="禁用" {
              disable-tunnel: w425 -> [w430 _]
              frame Disabled {
                n215 = Enqueue Element At Opposite End(queue=w430, element=cluster{"命令":string, "数据":variant} {"命令"="init", "数据"=variant} ("元素")) -> ()  [unwired: 2 in, 3 out]
              }
              frame Enabled {
              }
            }
            n216 = Wait (ms)(milliseconds to wait=u32 2000 ("等待时间（毫秒）")) -> ()  [unwired: 1 out]
          }
        }
        n217 = call <vilib>:"Clear Errors.vi"("error in (no error)"=w417) -> ("error out"=w416:errorcluster)  [unwired: 5 in, 1 out]
      }
    }
    n218 = Unbundle By Name(w199) -> ("status"=w197:bool)
    "通讯故障" <- w197
    n219 = global write "采配水全局变量.vi" "通讯故障"(w197) -> ()
  }
  n220 = property on="多列列表框" class="MCListbox (严格)"("ItemNames"=string[][] [["待机"], ["初始化"], ["水样润洗"], ["一级水样池进样"], ["二级水样池进样"], ["沉淀"], ["氨氮水样池进样"], ["配水"], ["反冲洗"], ["一级采样池储水"], ["结束"]] ("项名")) -> ()  [unwired: 2 in, 2 out]
  n221 = call-dynamic "Close Session.vi"("error in (no error)"=w8, "MB session in"=w7) -> ()  [unwired: 9 in, 1 out]
